vi "Log.vi"(8 "error in (no error)":errorcluster, 9 "Message":string, 10 "Level (info)":T1=enum."info", 11 "Facility":T2) -> (0 "error out":errorcluster)   [LabVIEW 2017, in "Log.lvclass"]
uses:
  Log.lvclass
  Log_Facilities.ctl
  Log_Level.ctl
  Log_Facility.ctl
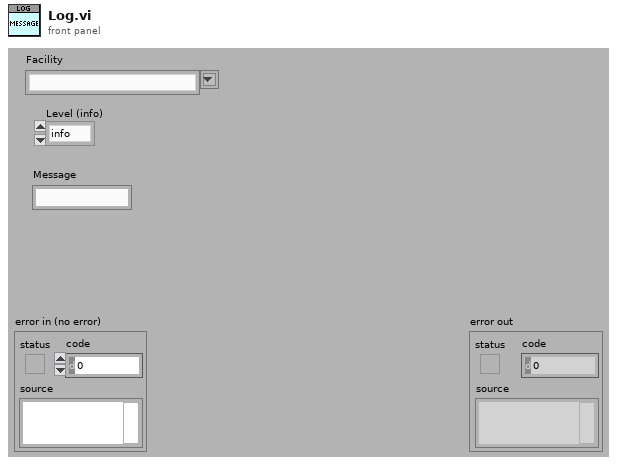
[diagram p1: front panel]
types:
  T1 = typedef "Log.lvclass/Log_Level.ctl" = enum16{"none", "info", "trace", "warn", "error", "fatal"}
  T2 = typedef "Log.lvclass/Log_Facilities.ctl" = string
  T3 = typedef "Log.lvclass/Log_Facility.ctl" = cluster{"Path":path, "Ref":refnum<file>, "Level":T1}
  T4 = typedef "Log.lvclass/ObjectAttributes.ctl" = cluster{"Level":T1, "Facilities":variant, "Event":refnum<user-event>}
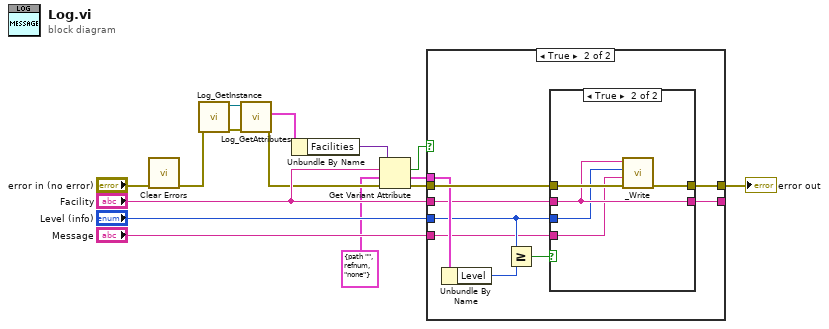
[diagram p0: block diagram]
diagram:
  n1 = call <vilib>:"Clear Errors.vi"("error in (no error)"="error in (no error)") -> ("error out"=w3:errorcluster)  [unwired: 5 in, 1 out]
  n2 = call "Log_GetInstance.vi"("error in (no error)"=w3) -> ("error out"=w12:errorcluster, "reference out"=w5:refnum<class "Log.lvclass">)  [unwired: 6 in, 3 out]
  n3 = call "Log_GetAttributes.vi"("error in (no error)"=w12, "reference in"=w5) -> ("error out"=w10:errorcluster, "Data"=w4:T4)  [unwired: 6 in, 2 out]
  n4 = Unbundle By Name(w4) -> ("Facilities"=w11:variant)
  n5 = Get Variant Attribute(Variant=w11, name="Facility", default value (empty Variant)=T3 {"Path"=path "", "Ref"=refnum, "Level"=enum."none"} ("Cluster"), error in=w10) -> (found=w6:bool, value=w8:T3, error out=w7:errorcluster)  [unwired: 1 out]
  n6 = case shown="True" w6 {
    tunnel: w8 -> [_ w23]
    tunnel: "Level (info)" -> [_ w20]
    tunnel: w7 -> [w17 w24]
    tunnel: [w17 w22] -> w1
    tunnel: "Facility" -> [w16 w21]
    tunnel: "Message" -> [_ w19]
    tunnel: [w16 w18] -> _
    frame False {
    }
    frame True {
      n7 = Unbundle By Name(w23) -> ("Level"=w26:T1)
      n8 = Greater Or Equal?(x=w20, y=w26) -> (x >= y?=w25:bool)
      n9 = case shown="True" w25 {
        tunnel: w24 -> [w28 w33]
        tunnel: [w28 w32] -> w22
        tunnel: w21 -> [w27 w31]
        tunnel: w20 -> [_ w29]
        tunnel: w19 -> [_ w30]
        tunnel: [w27 w31] -> w18
        frame False {
        }
        frame True {
          n10 = call "_Write.vi"("error in (no error)"=w33, "Message"=w30, "Level"=w29, "Name"=w31) -> ("error out"=w32:errorcluster)  [unwired: 7 in]
        }
      }
    }
  }
  "error out" <- w1
